vi "vipm_InstallPackagesbyPath.vi"(8 "error in (no error)":errorcluster, 11 "CommandLine":string[](array[string])) -> (0 "error out":errorcluster, 2 "test details":string, 3 "output to action":string)   [LabVIEW 2017]
uses:
  <vilib>/JKI/VIPM API/VIPM API_vipm_api.lvlib
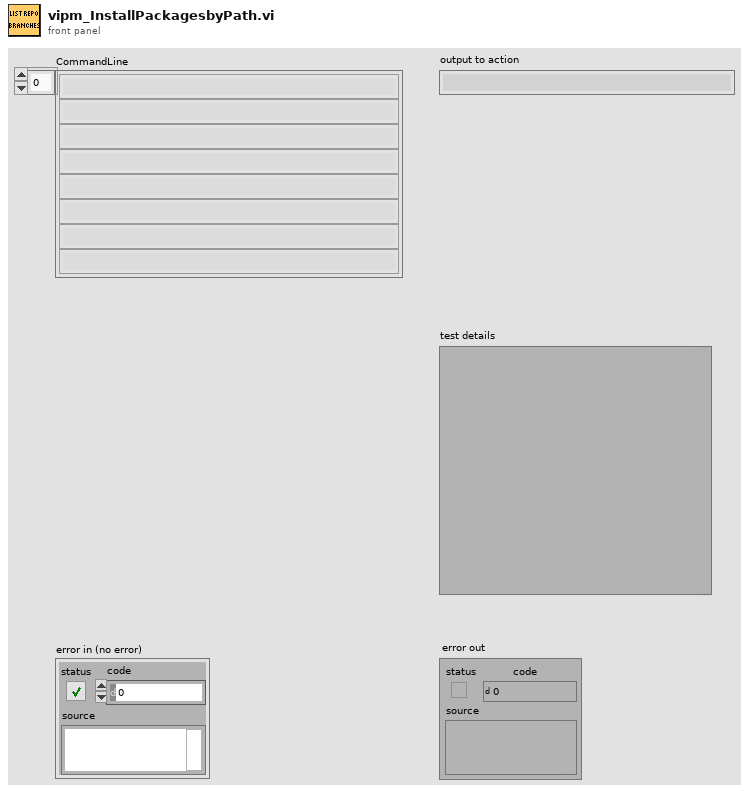
[diagram p1: front panel]
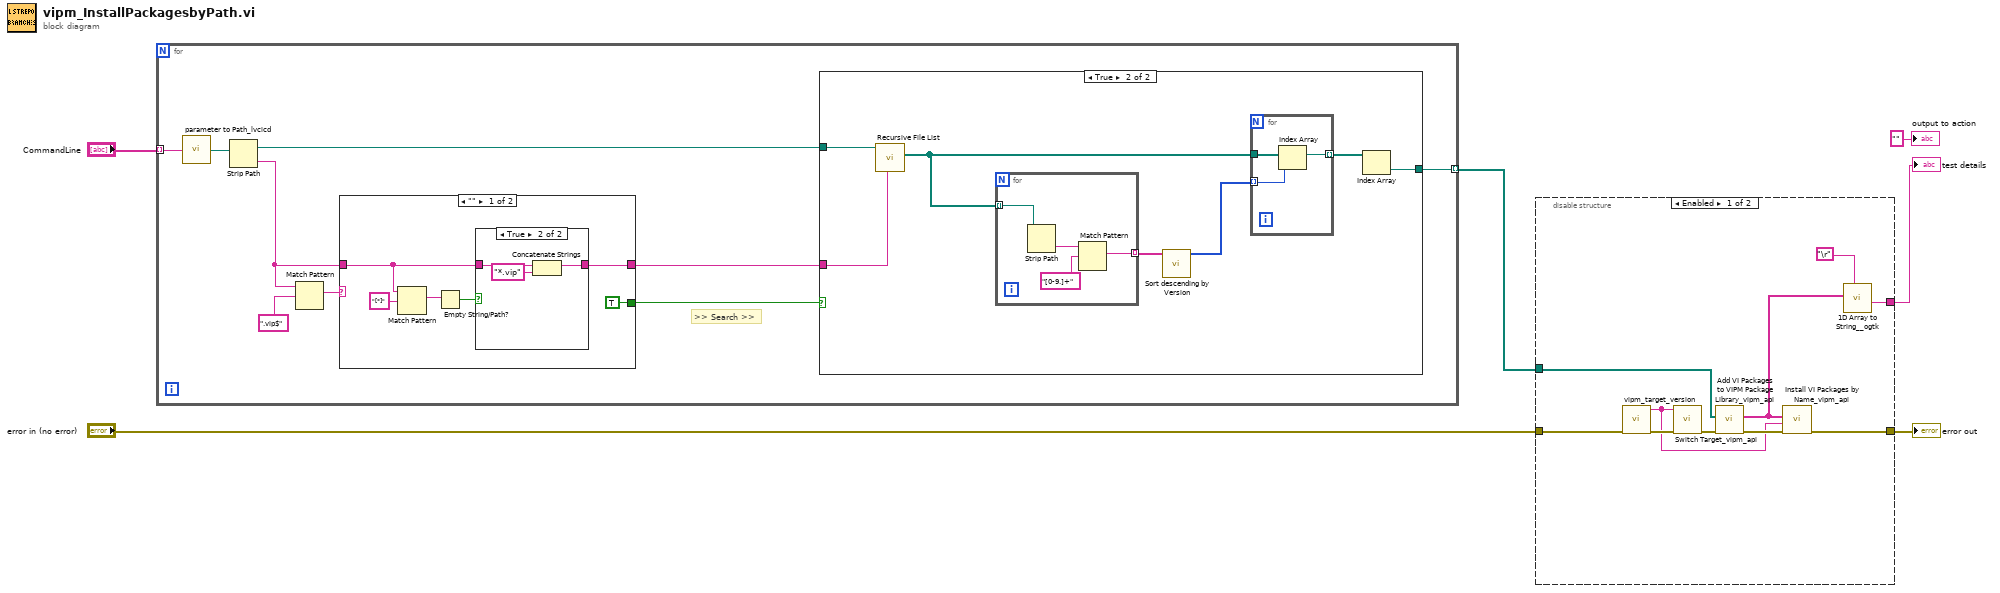
[diagram p0: block diagram]
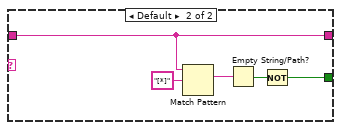
[diagram p5: hidden frame]
diagram:
  n1 = for {
    tunnel: [w12] -> w4 mode=indexing
    tunnel: "CommandLine" -> [w15] mode=indexing
    # ">> Search >>"
    n2 = call "parameter to Path_lvcicd.vi"("String"=w15) -> ("Path"=w14:path)
    n3 = Strip Path(path=w14) -> (stripped path=w13:path, name=w9:string)
    n4 = Match Pattern(string=w9, regular expression=".vip$") -> (match substring=w10:string)  [unwired: 1 in, 3 out]
    n5 = case shown="\"\"" w10 {
      tunnel: w9 -> [w31 w45]
      tunnel: [w32 w45] -> w8
      tunnel: [TRUE w41] -> w7
      frame "" {
        n6 = Match Pattern(string=w31, regular expression="[*]") -> (match substring=w35:string)  [unwired: 1 in, 3 out]
        n7 = Empty String/Path?(string/path=w35) -> (empty?=w34:bool)
        n8 = case shown="True" w34 {
          tunnel: [w37 w39] -> w32
          tunnel: w31 -> [w37 w40]
          frame False {
          }
          frame True {
            n9 = Concatenate Strings(w40, "*.vip" ("string")) -> (w39:string)
          }
        }
      }
      frame Default {
        n10 = Match Pattern(string=w45, regular expression="[*]") -> (match substring=w43:string)  [unwired: 1 in, 3 out]
        n11 = Empty String/Path?(string/path=w43) -> (empty?=w42:bool)
        n12 = Not(x=w42) -> (.not. x?=w41:bool)
      }
    }
    n13 = case shown="True" w7 {
      tunnel: w13 -> [w16 w23]
      tunnel: [w16 w22] -> w12
      tunnel: w8 -> [_ w19]
      frame False {
      }
      frame True {
        n14 = call <vilib>:"Recursive File List.vi"("pattern"=w19, "Folder Path"=w23) -> ("All Files in Dir"=w18:path[])  [unwired: 5 in, 4 out]
        n15 = for {
          tunnel: w18 -> [w25] mode=indexing
          tunnel: [w24] -> w17 mode=indexing
          n16 = Strip Path(path=w25) -> (name=w26:string)  [unwired: 1 out]
          n17 = Match Pattern(string=w26, regular expression="[0-9.]+") -> (match substring=w24:string)  [unwired: 1 in, 3 out]
        }
        n18 = call "Sort descending by Version.vi"("Array"=w17) -> ("Sorted Pointers"=w21:i32[])  [unwired: 10 in]
        n19 = for {
          tunnel: w18 -> [w30]
          tunnel: [w29] -> w20 mode=indexing
          tunnel: w21 -> [w28] mode=indexing
          n20 = Index Array(array=w30, index=w28) -> (element=w29:path)
        }
        n21 = Index Array(array=w20) -> (element=w22:path)  [unwired: 1 in]
      }
    }
  }
  n22 = disable-structure shown="Enabled" {
    disable-tunnel: [w53 _] -> w6
    disable-tunnel: w4 -> [w52 _]
    disable-tunnel: "error in (no error)" -> [w48 _]
    disable-tunnel: [w51 _] -> w2
    frame Enabled {
      n23 = call "vipm_target_version.vi"() -> ("vipm Taget version"=w46:string)  [unwired: 11 in]
      n24 = call <vilib>:"Switch Target_vipm_api.vi"("error in (no error)"=w48, "LabVIEW Version"=w46) -> ("error out"=w47:errorcluster)  [unwired: 9 in]
      n25 = call <vilib>:"Add VI Packages to VIPM Package Library_vipm_api.vi"("error in (no error)"=w47, "Packages to add to VIPM Library (vipc,vip,ogp)"=w52) -> ("error out"=w54:errorcluster, "Package Names Added"=w50:string[])  [unwired: 8 in]
      n26 = call <vilib>:"Install VI Packages by Name_vipm_api.vi"("error in (no error)"=w54, "LabVIEW Version"=w46, "Package Names to Install []"=w50) -> ("error out"=w53:errorcluster)  [unwired: 8 in]
      n27 = call <userlib>:"1D Array to String__ogtk.vi"("delimiter (Tab)"="\r", "Array of Strings"=w50) -> ("delimited string"=w51:string)  [unwired: 9 in]
    }
    frame Disabled {
    }
  }
  "test details" <- w2
  "error out" <- w6
  "output to action" <- "" ("output to action")
